vi "SR850.vi"(11 "error in":errorcluster) -> (0 "error out":errorcluster, 1 "Frequency":dbl, 2 "R":dbl, 3 "Theta":dbl)   [LabVIEW 2017, in "LD Reading.lvclass"]
uses:
  LD Reading.lvclass
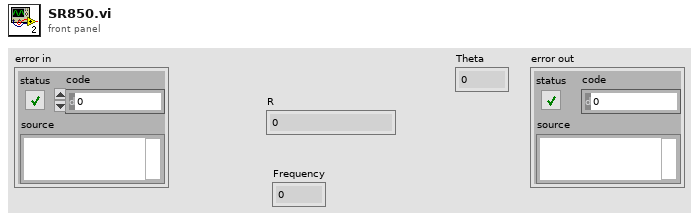
[diagram p1: front panel]
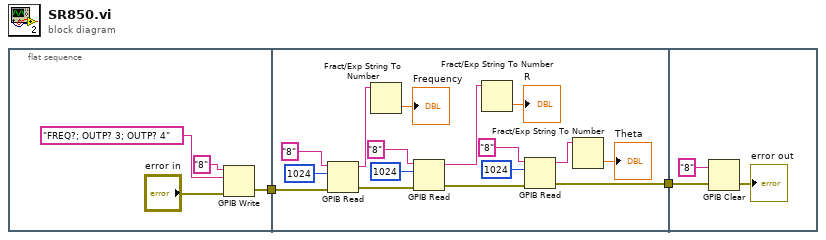
[diagram p0: block diagram]
diagram:
  n1 = flat-sequence {
    tunnel: [w4] -> w2
    tunnel: w2 -> [w22]
    tunnel: [w13] -> w1
    tunnel: w1 -> [w24]
    frame #0 {
      n2 = GPIB Write(0:"8" ("address string"), 1:"FREQ?; OUTP? 3; OUTP? 4" ("data"), 3:"error in") -> (6:w4:errorcluster)  [unwired: 2 in, 1 out]
    }
    frame #1 {
      n3 = GPIB Read(0:"8" ("address string"), 1:1024 ("byte count"), 3:w22) -> (5:w12:string, 7:w17:errorcluster)  [unwired: 2 in, 1 out]
      n4 = Fract/Exp String To Number(string=w12) -> (number=→"Frequency":dbl)  [unwired: 3 in, 1 out]
      n5 = GPIB Read(0:"8" ("address string"), 1:1024 ("byte count"), 3:w17) -> (5:w7:string, 7:w16:errorcluster)  [unwired: 2 in, 1 out]
      n6 = Fract/Exp String To Number(string=w7) -> (number=→"R":dbl)  [unwired: 3 in, 1 out]
      n7 = GPIB Read(0:"8" ("address string"), 1:1024 ("byte count"), 3:w16) -> (5:w11:string, 7:w13:errorcluster)  [unwired: 2 in, 1 out]
      n8 = Fract/Exp String To Number(string=w11) -> (number=→"Theta":dbl)  [unwired: 3 in, 1 out]
    }
    frame #2 {
      n9 = GPIB Clear(2:w24, 3:"8" ("address string")) -> (0:→"error out":errorcluster)  [unwired: 1 out]
    }
  }
